vi "InitializeOutputChannels.vi"(0 "AOTF":u16(ring) items=["None", "Laser 1", "Laser 2", "Laser 1 + 2", "Laser 3", "Laser 1 + 3", "Laser 2 + 3", "Laser 1+2+3", "Laser 1+2+3+4", "Laser 2+3+4"], 1 "1st Axis":u16(ring) items=["x", "y", "z", ""], 2 "Retrace":bool, 3 "EOM":u16(ring) items=["None", "Trace", "Retrace", "All"]) -> ()   [LabVIEW 2009]
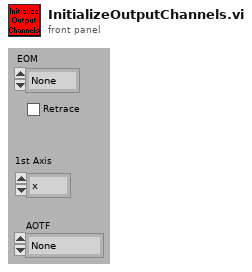
[diagram p1: front panel]
types:
  T1 = typedef "SPCConfiguration.ctt" = cluster{"SPC Initialization File":path, "Module Number":u16, "Operation Mode":u16, "Trigger Channel":tag}
  T2 = typedef "EOMSettings.ctt" = cluster{"Output Channel":tag, "EOM Voltage":dbl, "Pixel per Polymode Cycle":u32, "Time per Polymode Cycle":dbl}
  T3 = typedef "AOTFSettings.ctt" = cluster{"Laser 1 Output Channel":tag, "AOTF  1 Output Voltage":dbl, "Laser 2 Output Channel":tag, "AOTF  2 Output Voltage":dbl, "Laser 3 Output Channel":tag, "AOTF  3 Output Voltage":dbl, "Pixel per Cycle":u16, "Time per Cycle  / ms":dbl, "Laser 4 Output Channel":tag, "AOTF  4 Output Voltage":dbl}
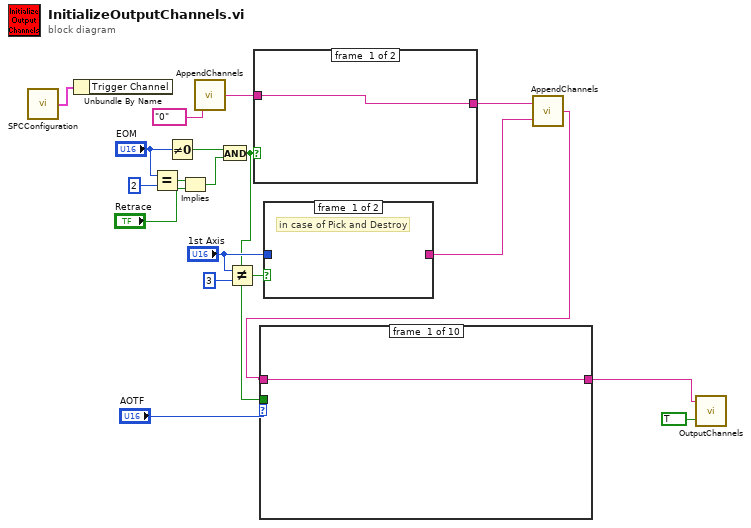
[diagram p0: block diagram]
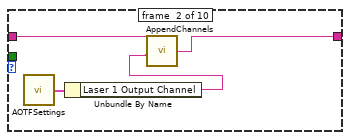
[diagram p2: hidden frame]
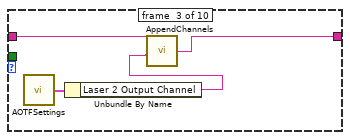
[diagram p3: hidden frame]
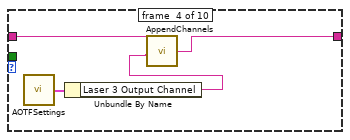
[diagram p4: hidden frame]
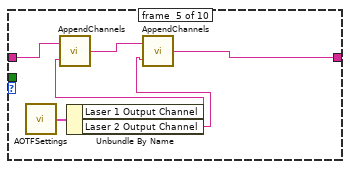
[diagram p5: hidden frame]
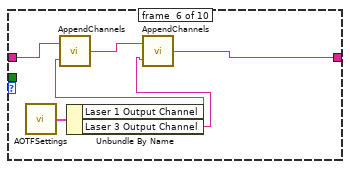
[diagram p6: hidden frame]
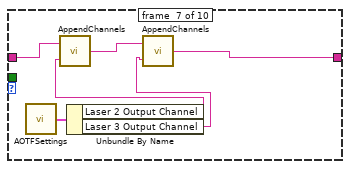
[diagram p7: hidden frame]
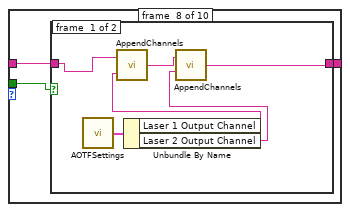
[diagram p8: hidden frame]
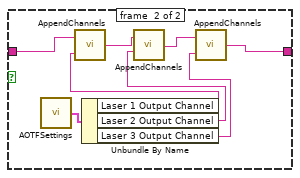
[diagram p9: hidden frame]
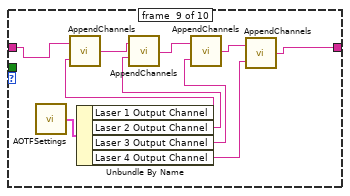
[diagram p10: hidden frame]
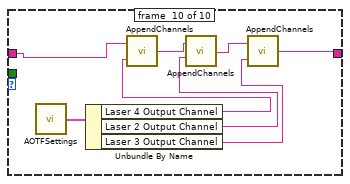
[diagram p11: hidden frame]
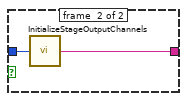
[diagram p12: hidden frame]
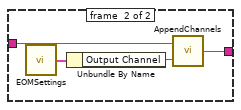
[diagram p13: hidden frame]
diagram:
  n1 = call "SPCConfiguration.vi"() -> ("SPC Configuration (output)"=w19:T1)  [unwired: 2 in]
  n2 = Unbundle By Name(w19) -> ()  [unwired: 1 out]
  n3 = Equal?(x="EOM", y=u16 2) -> (x = y?=w15:bool)
  n4 = Not Equal To 0?(x="EOM") -> (x != 0?=w18:bool)
  n5 = Implies(1:"Retrace", 2:w15) -> (0:w13:bool)
  n6 = call "AppendChannels.vi"("Append Channels"=tag "0") -> ("Output Channels (output)"=w12:tag)  [unwired: 1 in]
  n7 = And(x=w18, y=w13) -> (x .and. y?=w2:bool)
  n8 = Not Equal?(x="1st Axis", y=u16 3) -> (x != y?=w8:bool)
  n9 = case shown="True" w2 {
    tunnel: w12 -> [w20 w24]
    tunnel: [w20 w21] -> w11
    frame #0 {
    }
    frame #1 {
      n10 = call "EOMSettings.vi"() -> ("EOM Settings (output)"=w23:T2)  [unwired: 2 in]
      n11 = Unbundle By Name(w23) -> ("Output Channel"=w22:tag)
      n12 = call "AppendChannels.vi"("Append Channels"=w22, "Output Channels (input)"=w24) -> ("Output Channels (output)"=w21:tag)
    }
  }
  n13 = case shown="True" w8 {
    tunnel: "1st Axis" -> [_ w26]
    tunnel: [_ w25] -> w10
    frame #0 {
      # "in case of Pick and Destroy"
    }
    frame #1 {
      n14 = call "InitializeStageOutputChannels.vi"("1st Axis"=w26) -> ("Append Channels"=w25:tag)
    }
  }
  n15 = call "AppendChannels.vi"("Append Channels"=w10, "Output Channels (input)"=w11) -> ("Output Channels (output)"=w4:tag)
  n16 = case shown="9" "AOTF" {
    tunnel: w4 -> [w27 w31 w35 w39 w45 w51 w57 w60 w78 w86]
    tunnel: [w27 w30 w34 w38 w40 w46 w52 w59 w75 w85] -> w3
    tunnel: w2 -> [_ _ _ _ _ _ _ w58 _ _]
    frame #0 {
    }
    frame #1 {
      n17 = call "AOTFSettings.vi"() -> ("AOTF Setting (Output)"=w29:T3)  [unwired: 2 in]
      n18 = Unbundle By Name(w29) -> ("Laser 1 Output Channel"=w28:tag)
      n19 = call "AppendChannels.vi"("Append Channels"=w28, "Output Channels (input)"=w31) -> ("Output Channels (output)"=w30:tag)
    }
    frame #2 {
      n20 = call "AOTFSettings.vi"() -> ("AOTF Setting (Output)"=w33:T3)  [unwired: 2 in]
      n21 = Unbundle By Name(w33) -> ("Laser 2 Output Channel"=w32:tag)
      n22 = call "AppendChannels.vi"("Append Channels"=w32, "Output Channels (input)"=w35) -> ("Output Channels (output)"=w34:tag)
    }
    frame #3 {
      n23 = call "AOTFSettings.vi"() -> ("AOTF Setting (Output)"=w37:T3)  [unwired: 2 in]
      n24 = Unbundle By Name(w37) -> ("Laser 3 Output Channel"=w36:tag)
      n25 = call "AppendChannels.vi"("Append Channels"=w36, "Output Channels (input)"=w39) -> ("Output Channels (output)"=w38:tag)
    }
    frame #4 {
      n26 = call "AOTFSettings.vi"() -> ("AOTF Setting (Output)"=w44:T3)  [unwired: 2 in]
      n27 = Unbundle By Name(w44) -> ("Laser 1 Output Channel"=w43:tag, "Laser 2 Output Channel"=w41:tag)
      n28 = call "AppendChannels.vi"("Append Channels"=w43, "Output Channels (input)"=w45) -> ("Output Channels (output)"=w42:tag)
      n29 = call "AppendChannels.vi"("Append Channels"=w41, "Output Channels (input)"=w42) -> ("Output Channels (output)"=w40:tag)
    }
    frame #5 {
      n30 = call "AOTFSettings.vi"() -> ("AOTF Setting (Output)"=w50:T3)  [unwired: 2 in]
      n31 = Unbundle By Name(w50) -> ("Laser 1 Output Channel"=w49:tag, "Laser 3 Output Channel"=w47:tag)
      n32 = call "AppendChannels.vi"("Append Channels"=w49, "Output Channels (input)"=w51) -> ("Output Channels (output)"=w48:tag)
      n33 = call "AppendChannels.vi"("Append Channels"=w47, "Output Channels (input)"=w48) -> ("Output Channels (output)"=w46:tag)
    }
    frame #6 {
      n34 = call "AOTFSettings.vi"() -> ("AOTF Setting (Output)"=w56:T3)  [unwired: 2 in]
      n35 = Unbundle By Name(w56) -> ("Laser 2 Output Channel"=w55:tag, "Laser 3 Output Channel"=w53:tag)
      n36 = call "AppendChannels.vi"("Append Channels"=w55, "Output Channels (input)"=w57) -> ("Output Channels (output)"=w54:tag)
      n37 = call "AppendChannels.vi"("Append Channels"=w53, "Output Channels (input)"=w54) -> ("Output Channels (output)"=w52:tag)
    }
    frame #7 {
      n38 = case shown="False" w58 {
        tunnel: w60 -> [w66 w74]
        tunnel: [w65 w67] -> w59
        frame #0 {
          n39 = call "AOTFSettings.vi"() -> ("AOTF Setting (Output)"=w64:T3)  [unwired: 2 in]
          n40 = Unbundle By Name(w64) -> ("Laser 1 Output Channel"=w63:tag, "Laser 2 Output Channel"=w61:tag)
          n41 = call "AppendChannels.vi"("Append Channels"=w63, "Output Channels (input)"=w66) -> ("Output Channels (output)"=w62:tag)
          n42 = call "AppendChannels.vi"("Append Channels"=w61, "Output Channels (input)"=w62) -> ("Output Channels (output)"=w65:tag)
        }
        frame #1 {
          n43 = call "AOTFSettings.vi"() -> ("AOTF Setting (Output)"=w73:T3)  [unwired: 2 in]
          n44 = Unbundle By Name(w73) -> ("Laser 1 Output Channel"=w72:tag, "Laser 2 Output Channel"=w70:tag, "Laser 3 Output Channel"=w68:tag)
          n45 = call "AppendChannels.vi"("Append Channels"=w72, "Output Channels (input)"=w74) -> ("Output Channels (output)"=w71:tag)
          n46 = call "AppendChannels.vi"("Append Channels"=w70, "Output Channels (input)"=w71) -> ("Output Channels (output)"=w69:tag)
          n47 = call "AppendChannels.vi"("Append Channels"=w68, "Output Channels (input)"=w69) -> ("Output Channels (output)"=w67:tag)
        }
      }
    }
    frame #8 {
      n48 = call "AOTFSettings.vi"() -> ("AOTF Setting (Output)"=w79:T3)  [unwired: 2 in]
      n49 = Unbundle By Name(w79) -> ("Laser 1 Output Channel"=w80:tag, "Laser 2 Output Channel"=w82:tag, "Laser 3 Output Channel"=w84:tag, "Laser 4 Output Channel"=w76:tag)
      n50 = call "AppendChannels.vi"("Append Channels"=w80, "Output Channels (input)"=w78) -> ("Output Channels (output)"=w81:tag)
      n51 = call "AppendChannels.vi"("Append Channels"=w82, "Output Channels (input)"=w81) -> ("Output Channels (output)"=w83:tag)
      n52 = call "AppendChannels.vi"("Append Channels"=w84, "Output Channels (input)"=w83) -> ("Output Channels (output)"=w77:tag)
      n53 = call "AppendChannels.vi"("Append Channels"=w76, "Output Channels (input)"=w77) -> ("Output Channels (output)"=w75:tag)
    }
    frame #9 {
      n54 = call "AOTFSettings.vi"() -> ("AOTF Setting (Output)"=w87:T3)  [unwired: 2 in]
      n55 = Unbundle By Name(w87) -> ("Laser 4 Output Channel"=w88:tag, "Laser 2 Output Channel"=w90:tag, "Laser 3 Output Channel"=w92:tag)
      n56 = call "AppendChannels.vi"("Append Channels"=w88, "Output Channels (input)"=w86) -> ("Output Channels (output)"=w89:tag)
      n57 = call "AppendChannels.vi"("Append Channels"=w90, "Output Channels (input)"=w89) -> ("Output Channels (output)"=w91:tag)
      n58 = call "AppendChannels.vi"("Append Channels"=w92, "Output Channels (input)"=w91) -> ("Output Channels (output)"=w85:tag)
    }
  }
  n59 = call "OutputChannels.vi"("Get/Set"=TRUE, "Output Channels (input)"=w3) -> ()  [unwired: 1 out]
